vi "fileNameCreator.vi"(10 "folder":string, 11 "Measurement ID":string) -> (3 "concatenated string":string)   [LabVIEW 2009]
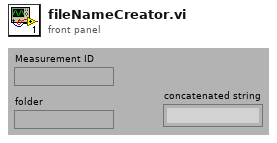
[diagram p1: front panel]
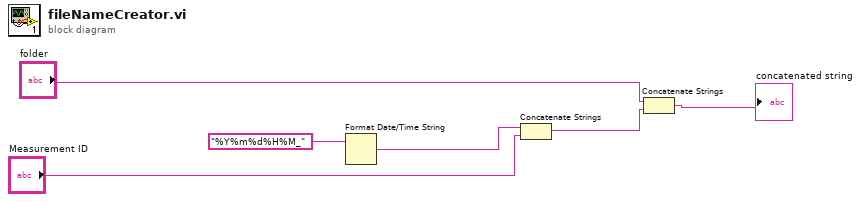
[diagram p0: block diagram]
diagram:
  n1 = Format Date/Time String(time format string (%c)="%Y%m%d%H%M_") -> (date/time string=w5:string)  [unwired: 2 in]
  n2 = Concatenate Strings(w5, "Measurement ID") -> (w3:string)
  n3 = Concatenate Strings("folder", w3) -> (→"concatenated string":string)
